vi "DELETE Sum Input Channel.vi"   [LabVIEW 2013]
uses:
  Action.ctl
  Channel FGV Selector.ctl
types:
  T1 = typedef "Channel FGV Selector.ctl" = enum16{"Division Input", "Sum Input", "Z Output", "Z Input", "Y Output", "Y Input", "X Output", "X Input"}
  T2 = typedef "Action.ctl" = enum16{"GET", "PUT", "DELETE"}
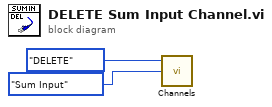
[diagram p0: block diagram]
diagram:
  n1 = call "Channels.vi"("Channel FGV Selector"=Channel_FGV_Selector."Sum Input", "Action"=Action."DELETE") -> ()  [unwired: 1 in, 1 out]
